vi "Read_Selected_channels.vi"(1 "Valid Channel Options":string[][](array[string]), 2 "Template Names":string[](array[string]), 3 "Data string":string, 5 "All Channels Present":string[](array[string]), 7 "Extra Channels":string[][](array[string]), 12 "Filetype":string, 14 "Ignore When":string[][](array[string])) -> (4 "Non-Blank Rows":i32[](array[numeric]), 8 "Deleted Rows":string[][](array[string]), 10 "Output Values":string[][](array[string]))   [LabVIEW 2021]
panel:
  out "Case":string
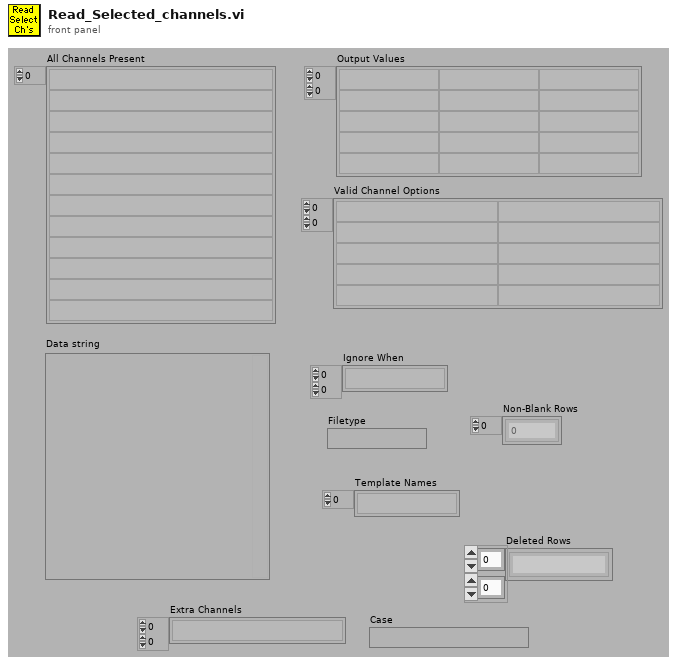
[diagram p1: front panel]
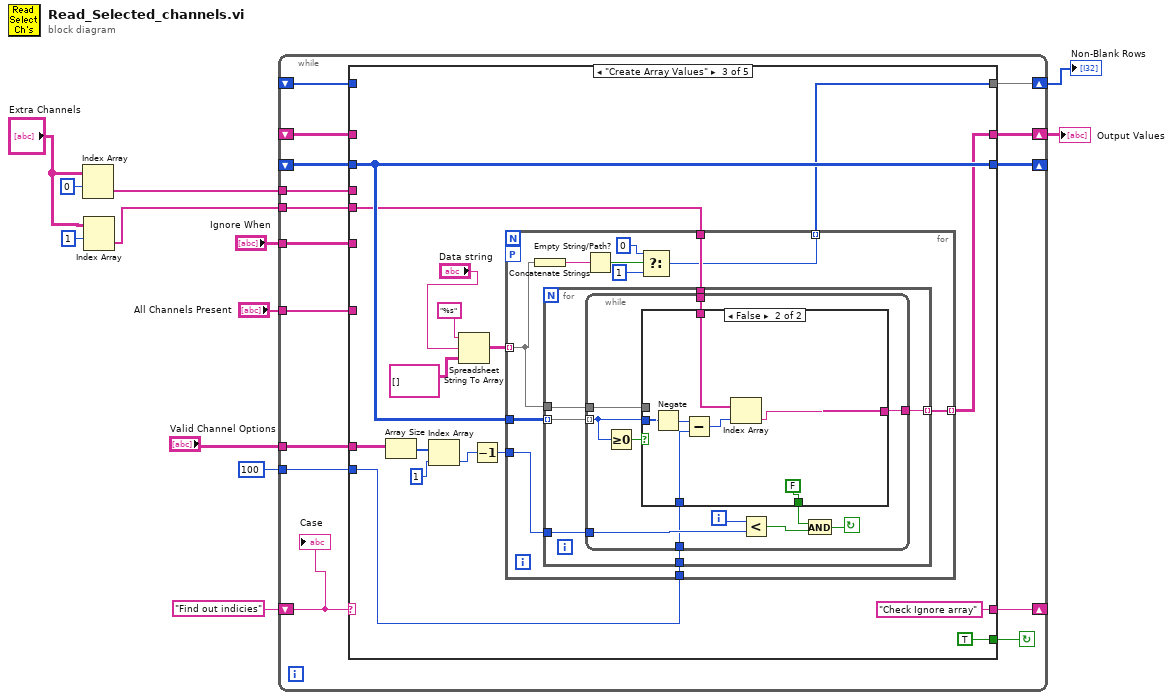
[diagram p0: block diagram]
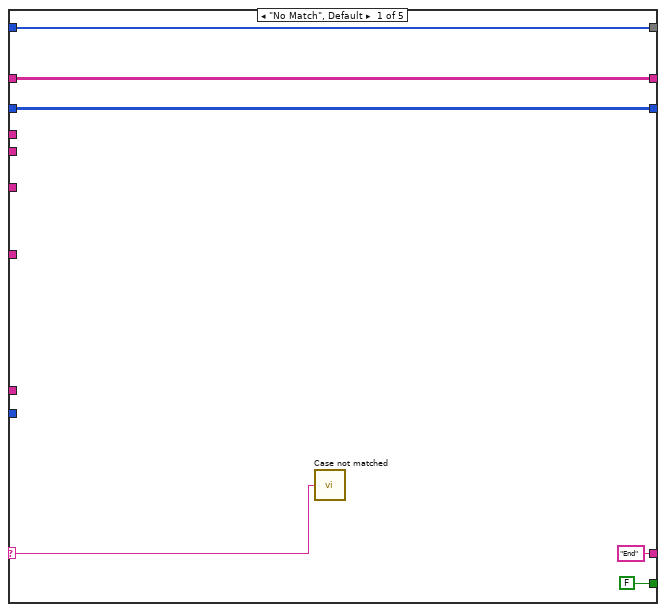
[diagram p2: hidden frame]
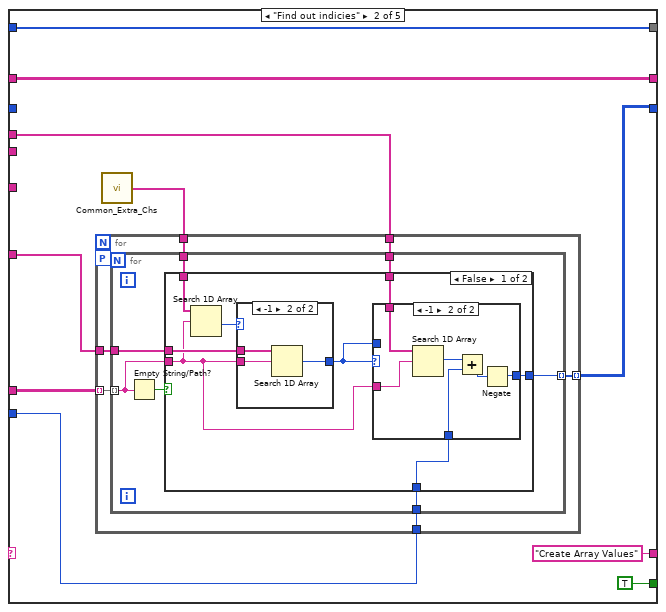
[diagram p3: hidden frame]
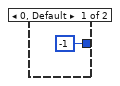
[diagram p4: hidden frame]
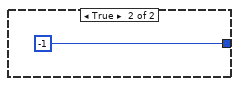
[diagram p6: hidden frame]
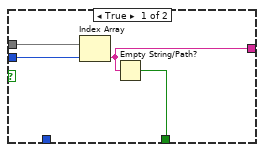
[diagram p7: hidden frame]
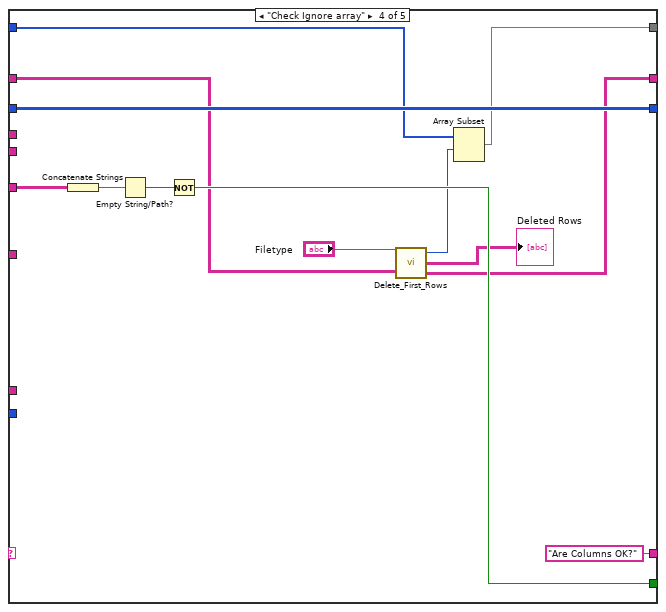
[diagram p8: hidden frame]
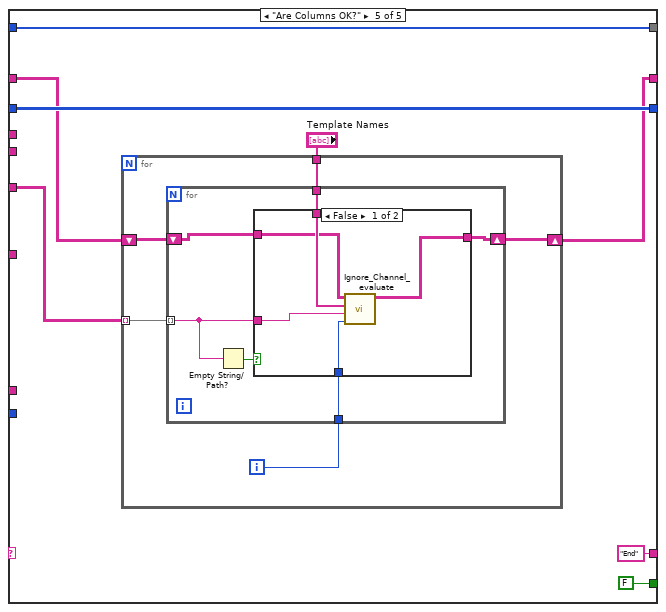
[diagram p9: hidden frame]
diagram:
  n1 = Index Array(array="Extra Channels", index (row)=0) -> (element=w1:string[])  [unwired: 1 in]
  n2 = Index Array(array="Extra Channels", index (row)=1) -> (element=w2:string[])  [unwired: 1 in]
  n3 = while {
    tunnel: "Ignore When" -> [w17]
    shift-left: _ -> [w18]
    shift-right: [w19] -> w8
    tunnel: 100 ("y") -> [w20]
    tunnel: "Valid Channel Options" -> [w21]
    tunnel: "All Channels Present" -> [w22]
    shift-left: _ -> [w24]
    shift-right: [w23] -> _
    shift-left: "Find out indicies" -> [w26]
    shift-right: [w25] -> _
    shift-right: [w16] -> w6
    shift-left: _ -> [w15]
    tunnel: w2 -> [w14]
    tunnel: w1 -> [w13]
    stop <- w27 continue-if-true
    n4 = case shown="\"Create Array Values\"" w26 {
      selector: w26 -> [w28 _ _ _ _]
      tunnel: [FALSE ("Results File?") TRUE ("Results File?") TRUE ("Results File?") w139 FALSE ("Results File?")] -> w27
      tunnel: ["End" "Create Array Values" ("f") "Check Ignore array" ("f") "Are Columns OK?" "End"] -> w25
      tunnel: w24 -> [w31 _ w84 w143 w151]
      tunnel: [w31 w39 w84 w143 w151] -> w23
      tunnel: w22 -> [_ w40 _ _ _]
      tunnel: w21 -> [_ w41 w86 _ _]
      tunnel: w20 -> [_ w38 w90 _ _]
      tunnel: [w30 w37 w80 w137 w145] -> w19
      tunnel: w18 -> [w30 w37 _ w136 w146]
      tunnel: w17 -> [_ _ _ w142 w149]
      tunnel: [w29 w36 w79 w133 w147] -> w16
      tunnel: w15 -> [w29 w36 _ w134 w147]
      tunnel: w14 -> [_ _ w78 _ _]
      tunnel: w13 -> [_ w34 _ _ _]
      frame "No Match", Default {
        n5 = call "Case not matched.vi"("Case Name not Matched"=w28) -> ()
      }
      frame "Find out indicies" {
        n6 = call "Common_Extra_Chs.vi"() -> ("Common Extra Channels"=w35:string[])
        n7 = for {
          tunnel: w40 -> [w49]
          tunnel: w41 -> [w48] mode=indexing
          tunnel: [w47] -> w39 mode=indexing
          tunnel: w38 -> [w46]
          tunnel: w34 -> [w45]
          tunnel: w35 -> [w44]
          workers-P: _ -> [_]
          n8 = for {
            tunnel: w48 -> [w54] mode=indexing
            tunnel: w49 -> [w56]
            tunnel: [w55] -> w47 mode=indexing
            tunnel: w46 -> [w52]
            tunnel: w45 -> [w51]
            tunnel: w44 -> [w50]
            n9 = Empty String/Path?(string/path=w54) -> (empty?=w53:bool)
            n10 = case shown="False" w53 {
              tunnel: w56 -> [w64 _]
              tunnel: [w63 -1 ("index of element")] -> w55
              tunnel: w54 -> [w58 _]
              tunnel: w52 -> [w61 _]
              tunnel: w51 -> [w60 _]
              tunnel: w50 -> [w59 _]
              frame False {
                n11 = Search 1D Array(1D array=w59, element=w58) -> (index of element=w57:i32)  [unwired: 1 out]
                n12 = case shown="-1" w57 {
                  tunnel: w64 -> [_ w68]
                  tunnel: [-1 ("index of element") w67] -> w62
                  tunnel: w58 -> [_ w66]
                  frame 0, Default {
                  }
                  frame -1 {
                    n13 = Search 1D Array(1D array=w68, element=w66) -> (index of element=w67:i32)  [unwired: 1 out]
                  }
                }
                n14 = case shown="-1" w62 {
                  tunnel: w58 -> [_ w75]
                  tunnel: [w69 w72] -> w63
                  tunnel: w62 -> [w69 _]
                  tunnel: w61 -> [_ w71]
                  tunnel: w60 -> [_ w70]
                  frame 0, Default {
                  }
                  frame -1 {
                    n15 = Search 1D Array(1D array=w70, element=w75) -> (index of element=w74:i32)  [unwired: 1 out]
                    n16 = Add(x=w74, y=w71) -> (x+y=w73:i32)
                    n17 = Negate(x=w73) -> (-x=w72:i32)
                  }
                }
              }
              frame True {
              }
            }
          }
        }
      }
      frame "Create Array Values" {
        n18 = Array Size(array=w86) -> (size(s)=w89:i32[])
        n19 = Index Array(array=w89, index=1 ("Index")) -> (element=w87:i32)
        n20 = Spreadsheet String To Array(format string="%s", spreadsheet string="Data string", array type (2D Dbl)=string[][] []) -> (array=w81:string[][])  [unwired: 1 out]
        n21 = Decrement(x=w87) -> (x-1=w85:i32)
        n22 = for {
          tunnel: w84 -> [w103]
          tunnel: w81 -> [w97] mode=indexing
          tunnel: [w102] -> w80 mode=indexing
          tunnel: w90 -> [w101]
          tunnel: w78 -> [w100]
          tunnel: w85 -> [w99]
          tunnel: [w95] -> w79 mode=indexing
          workers-P: _ -> [_]
          n23 = Concatenate Strings(w97) -> (w98:string)
          n24 = for {
            tunnel: w103 -> [w107] mode=indexing
            tunnel: w97 -> [w109]
            tunnel: [w108] -> w102 mode=indexing
            tunnel: w99 -> [w106]
            tunnel: w101 -> [w105]
            tunnel: w100 -> [w104]
            n25 = while {
              tunnel: w104 -> [w110]
              tunnel: w105 -> [w111]
              tunnel: w106 -> [w117]
              tunnel: w107 -> [w113] mode=indexing
              tunnel: [w119] -> w108
              tunnel: w109 -> [w120]
              i -> [w118]
              stop <- w115 continue-if-true
              n26 = Greater Or Equal To 0?(x=w113) -> (x >= 0?=w112:bool)
              n27 = case shown="False" w112 {
                tunnel: w120 -> [w124 _]
                tunnel: [w122 w131] -> w119
                tunnel: w113 -> [w123 w130]
                tunnel: [w121 FALSE] -> w114
                tunnel: w111 -> [_ w128]
                tunnel: w110 -> [_ w125]
                frame True {
                  n28 = Index Array(array=w124, index=w123) -> (element=w122:string)
                  n29 = Empty String/Path?(string/path=w122) -> (empty?=w121:bool)
                }
                frame False {
                  n30 = Negate(x=w130) -> (-x=w129:i32)
                  n31 = Subtract(x=w129, y=w128) -> (x-y=w127:i32)
                  n32 = Index Array(array=w125, index=w127) -> (element=w131:string)
                }
              }
              n33 = Less?(x=w118, y=w117) -> (x < y?=w116:bool)
              n34 = And(x=w114, y=w116) -> (x .and. y?=w115:bool)
            }
          }
          n35 = Empty String/Path?(string/path=w98) -> (empty?=w96:bool)
          n36 = Select(t=0, s=w96, f=1) -> (s? t:f=w95:i32)
        }
      }
      frame "Check Ignore array" {
        n37 = Concatenate Strings(w142) -> (w141:string)
        n38 = Empty String/Path?(string/path=w141) -> (empty?=w140:bool)
        n39 = Not(x=w140) -> (.not. x?=w139:bool)
        n40 = call "Delete_First_Rows.vi"("File Type (Default: AutoTrim)"="Filetype", "Data In"=w136) -> ("Rows removed"=w135:i32, "Deleted Rows"=→"Deleted Rows":string[][], "Data Out"=w137:string[][])
        n41 = Array Subset(array=w134, index=w135) -> (w133:i32[])  [unwired: 1 in]
      }
      frame "Are Columns OK?" {
        n42 = for {
          tunnel: "Template Names" -> [w157]
          tunnel: w149 -> [w156] mode=indexing
          shift-right: [w155] -> w145
          shift-left: w146 -> [w154]
          i -> [w153]
          n43 = for {
            tunnel: w157 -> [w163]
            tunnel: w156 -> [w161] mode=indexing
            shift-right: [w160] -> w155
            shift-left: w154 -> [w159]
            tunnel: w153 -> [w158]
            n44 = Empty String/Path?(string/path=w161) -> (empty?=w162:bool)
            n45 = case shown="False" w162 {
              tunnel: w163 -> [w168 _]
              tunnel: w161 -> [w167 _]
              tunnel: [w166 w169] -> w160
              tunnel: w159 -> [w165 w169]
              tunnel: w158 -> [w164 _]
              frame False {
                n46 = call "Ignore_Channel_evaluate.vi"("Column Index"=w164, "Ignore When String"=w167, "Template Names"=w168, "Data"=w165) -> ("Data Out"=w166:string[][])  [unwired: 3 in]
              }
              frame True {
              }
            }
          }
        }
      }
    }
    "Case" <- w26
  }
  "Output Values" <- w8
  "Non-Blank Rows" <- w6
